vi "prueba 1 repechaje.vi"() -> ()   [LabVIEW 2026]
panel:
  out "Voltaje Bajo":bool
  out "Voltaje Medio":bool
  out "Voltaje Normal":bool
  in  "stop":bool
  out "Voltaje V":dbl(knob) scale=0.0..3.3
  out "Humedad %":dbl(slide) scale=0.0..100.0
  out "Temperatura °C":dbl(slide) scale=0.0..100.0
  out "dato recibido":string
  # "Sistema de monitoreo De Mataplantas"
  # "Integrantes: Nilson Ayala \n                      Melissa Rojas\n                      Francisco Muñoz"
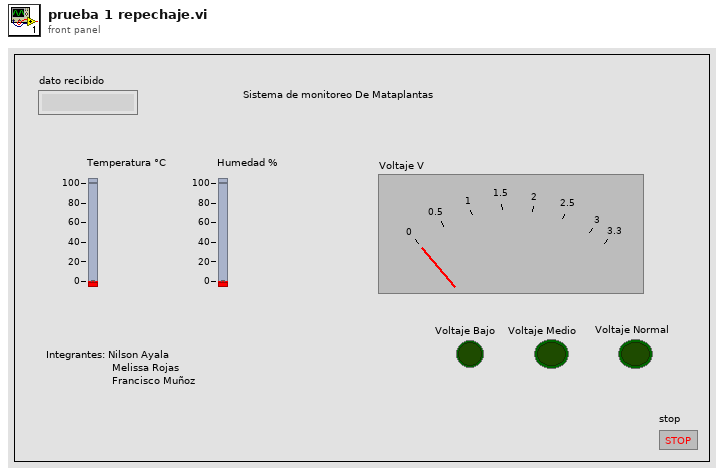
[diagram p1: front panel]
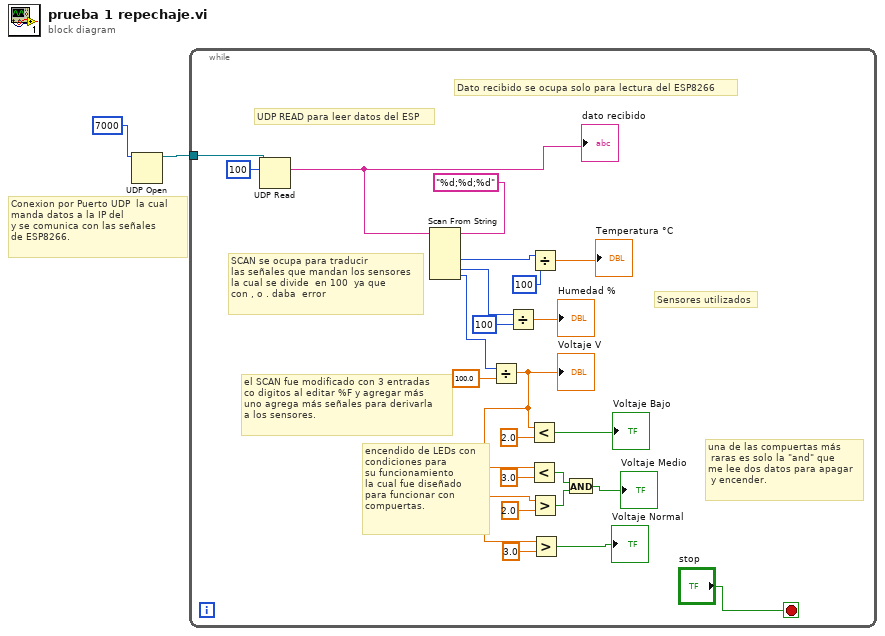
[diagram p0: block diagram]
diagram:
  # "Conexion por Puerto UDP  la cual\nmanda datos a la IP del\ny se comunica con las señales\nde ESP8266."
  n1 = UDP Open(11:u32 7000 ("net address")) -> (port=w1:refnum<k16>)  [unwired: 4 in, 2 out]
  n2 = while {
    tunnel: w1 -> [w23]
    stop <- "stop" stop-if-true
    # "el SCAN fue modificado con 3 entradas\nco digitos al editar %F y agregar más \nuno agrega más señales para derivarla \na los sensores."
    # "una de las compuertas más\n raras es solo la \"and\" que \nme lee dos datos para apagar\n y encender."
    # "encendido de LEDs con\ncondiciones para\nsu funcionamiento \nla cual fue diseñado \npara funcionar con \ncompuertas."
    # "Sensores utilizados"
    # "SCAN se ocupa para traducir \nlas señales que mandan los sensores\nla cual se divide  en 100  ya que\ncon , o . daba  error"
    # "UDP READ para leer datos del ESP"
    # "Dato recibido se ocupa solo para lectura del ESP8266"
    n3 = UDP Read(connection ID=w23, max size (548)=100) -> (data out=w21:string)  [unwired: 2 in, 4 out]
    "dato recibido" <- w21
    n4 = Scan From String "Scan From String"(format string="%d;%d;%d", input string=w21) -> (output 1=w20:i32, output 2=w16:i32, output 3=w13:i32)  [unwired: 5 in, 3 out]
    n5 = Divide(x=w13, y=100.0) -> (x/y=w3:dbl)
    "Voltaje V" <- w3
    n6 = Divide(x=w16, y=100) -> (x/y=→"Humedad %":dbl)
    n7 = Less?(x=w3, y=2.0) -> (x < y?=→"Voltaje Bajo":bool)
    n8 = Less?(x=w3, y=3.0) -> (x < y?=w8:bool)
    n9 = Divide(x=w20, y=100) -> (x/y=→"Temperatura °C":dbl)
    n10 = Greater?(x=w3, y=2.0) -> (0:w4:bool)
    n11 = Greater?(x=w3, y=3.0) -> (0:→"Voltaje Normal":bool)
    n12 = And(x=w8, y=w4) -> (x .and. y?=→"Voltaje Medio":bool)
  }
